vi "Adjust Shooter.vi"(6 "Upside Down?":bool, 7 "Start to Adjust":bool) -> (0 "Second Cannon":dbl, 1 "First Cannon":dbl, 2 "Cannon Angle":dbl, 3 "READY!":bool)   [LabVIEW 2012]
uses:
  BotStatus.vi
  <vilib>/express/express arith-compare/Formula/XNode/ExpressFormulaBlockNode.xnode
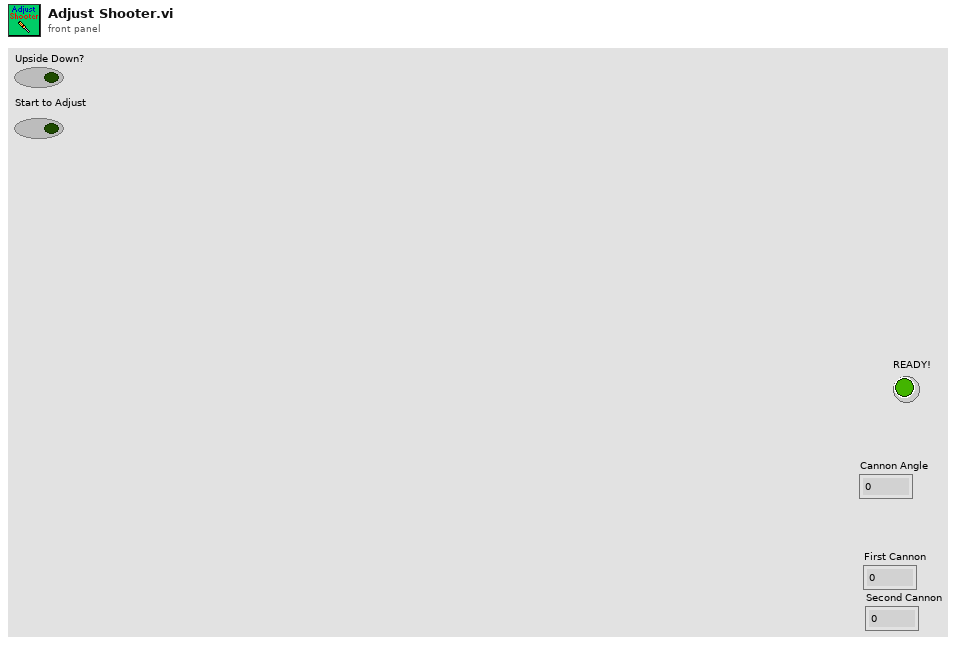
[diagram p1: front panel]
types:
  T1 = typedef "WPI_EncoderDevRef.ctl" = cluster{"DevStatus":errorcluster, "EncoderIndex":T2, "CounterIndex":T3, "DistancePerCount":dbl, "Decoding Type":T4}
  T2 = typedef "FPGA_EncoderIdx.ctl" = enum8{"Enc 0", "Enc 1", "Enc 2", "Enc 3", "Invalid"}
  T3 = typedef "FPGA_CounterCtrSystemIndex.ctl" = enum8{"Ctr 0", "Ctr 1", "Ctr 2", "Ctr 3", "Ctr 4", "Ctr 5", "Ctr 6", "Ctr 7", "Invalid"}
  T4 = typedef "WPI_EncoderType.ctl" = enum16{"1x", "2x", "4x"}
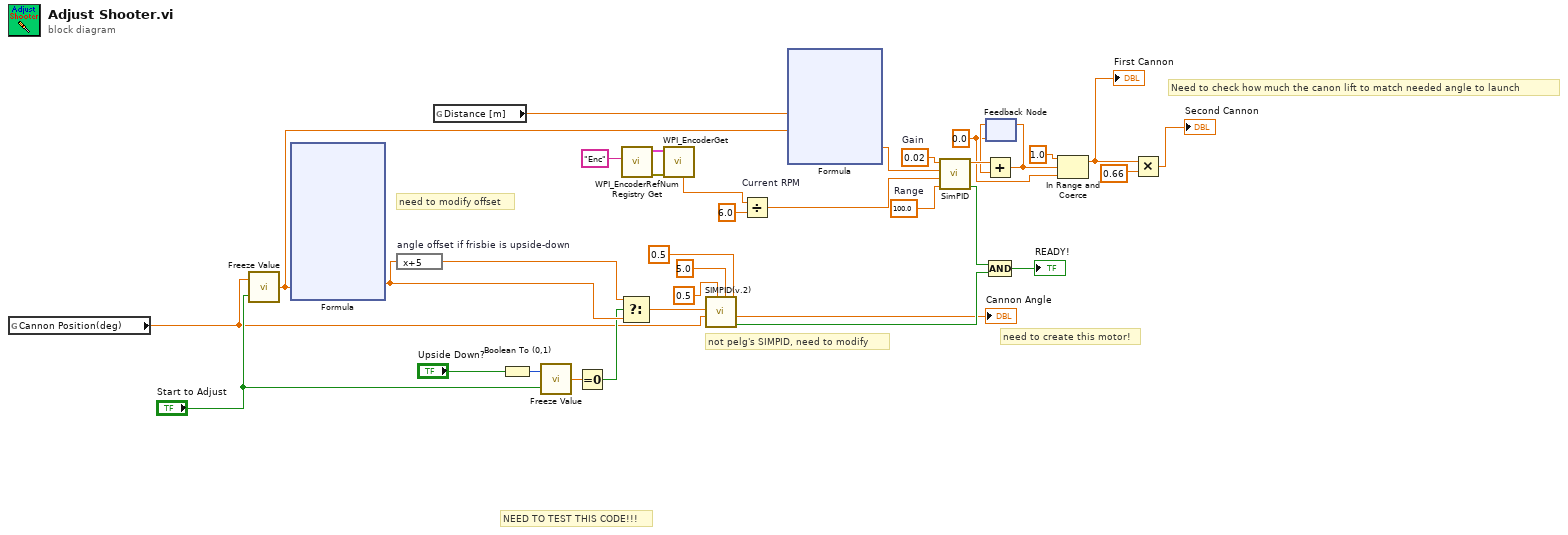
[diagram p0: block diagram]
diagram:
  w12 = 0.0
  w21 = 100.0  # Range
  w22 = 0.02  # Gain
  # "NEED TO TEST THIS CODE!!!"
  # "Need to check how much the canon lift to match needed angle to launch"
  # "need to create this motor!"
  # "need to modify offset"
  # "not pelg's SIMPID, need to modify"
  n1 = global read "BotStatus.vi" "Cannon Position(deg)"() -> (w2:dbl)
  n2 = call "Freeze Value.vi"("Freeze Value"="Start to Adjust", "In Value"=w2) -> ("Value Out"=w8:dbl)
  n3 = xnode "Formula"("angle"=w8) -> ("Result"=w10:dbl)  [unwired: 4 in, 1 out]
  n4 = expression code="x+5" "angle offset if frisbie is upside-down"(w10) -> (w9:dbl)
  n5 = global read "BotStatus.vi" "Distance [m]"() -> (w1:dbl)
  n6 = Boolean To (0,1)(Boolean="Upside Down?") -> (0, 1=w5:i16)
  n7 = call "Freeze Value.vi"("Freeze Value"="Start to Adjust", "In Value"=w5) -> ("Value Out"=w4:dbl)
  n8 = Equal To 0?(x=w4) -> (x = 0?=w3:bool)
  n9 = Select(t=w9, s=w3, f=w10) -> (s? t:f=w11:dbl)
  n10 = call <vilib>:"WPI_EncoderRefNum Registry Get.vi"("refnum name"="Enc") -> ("error out"=w27:errorcluster, "EncoderDevRef"=w28:T1)  [unwired: 9 in]
  n11 = call <vilib>:"WPI_EncoderGet.vi"("error in (no error)"=w27, "EncoderDevRef"=w28) -> ("Rate"=w25:dbl)  [unwired: 4 in, 5 out]
  n12 = call "SIMPID(v.2).vi"("Range"=0.5, "upper limit"=5.0, "lower limit"=0.5, "Current Point"=w2, "Set Point"=w11) -> ("On Target"=w32:bool, "result"=→"Cannon Angle":dbl)  [unwired: 5 in]
  n13 = Divide "Current RPM"(x=w25, y=6.0) -> (x/y=w20:dbl)
  n14 = xnode "Formula"("D"=w1, "angle"=w8) -> ("Result"=w19:dbl)  [unwired: 1 in, 1 out]
  n15 = call "SimPID.vi"("Range"=w21, "Position"=w20, "Set Point"=w19, "Gain"=w22) -> ("On Target"=w18:bool, "result"=w17:dbl)  [unwired: 5 in]
  n16 = feedback #1(w12) -> (w16:dbl)
  n17 = Add(x=w17, y=w16) -> (x+y=w15:dbl)
  n18 = feedback-in #1(w15) -> ()
  n19 = Compound Arithmetic op=AND(w18, w32) -> (→"READY!":bool)
  n20 = In Range and Coerce(upper limit=1.0, x=w15, lower limit=w12) -> (coerced(x)=w14:dbl)  [unwired: 1 out]
  "First Cannon" <- w14
  n21 = Multiply(x=w14, y=0.66) -> (x*y=→"Second Cannon":dbl)
